vi "Teleop.vi"(10 "Match Info":T1={"Autonomous Elapsed Seconds"=0.0, "TeleOp Elapsed Seconds"=0.0, "Disabled Elapsed Seconds"=0.0, "Visited Autonomous"=FALSE, "Visited TeleOp"=FALSE, "Visited Disabled"=FALSE, "Autonomous Settings"={"Autonomous Style"=enum."Independent", "VI Refnum"=refnum}}, 11 "Call Context":T2) -> ()   [LabVIEW 2013]
doc: "This VI is called for each TeleOp packet received from the DS where the robot is not disabled. It is often used to read from the joysticks and update I/O or to update setpoints for timed control loops. It should complete and return within 20 milliseconds or it may miss DS packets."
uses:
  Robot Global Data.vi
  <vilib>/Rock Robotics/WPI/DriverStation/DriverStationLCD/WPI_DriverStationLCDLCDLine.ctl
  <vilib>/Rock Robotics/WPI/RobotDrive/WPI_RobotDriveArcadeDrive_Standard(NoSaturation).vi
  <vilib>/Rock Robotics/WPI/Solenoid/Deprecated/WPI_SolenoidSetBool.vi
  <vilib>/Rock Robotics/WPI/DriverStation/WPI_DriverStationMatch Info.ctl
  <vilib>/Rock Robotics/WPI/DriverStation/WPI_DriverStationDerivedRobotMode.ctl
panel:
  out "Numeric 1":dbl(slide) scale=0.0..100.0
  out "Boolean 2":bool
  out "Boolean 1":bool
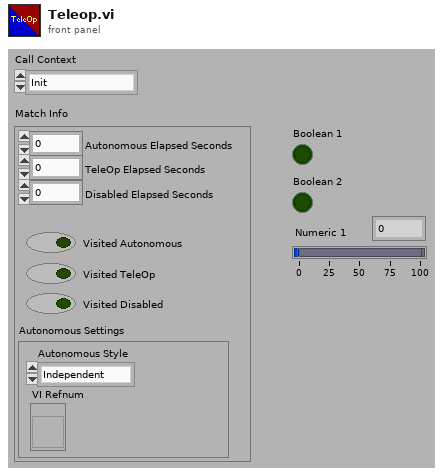
[diagram p1: front panel]
types:
  T1 = typedef "WPI_DriverStationMatch Info.ctl" = cluster{"Autonomous Elapsed Seconds":dbl, "TeleOp Elapsed Seconds":dbl, "Disabled Elapsed Seconds":dbl, "Visited Autonomous":bool, "Visited TeleOp":bool, "Visited Disabled":bool, "Autonomous Settings":cluster{"Autonomous Style":enum16{"Iterative", "Independent"}, "VI Refnum":refnum<vi>}}
  T2 = typedef "WPI_DriverStationDerivedRobotMode.ctl" = enum16{"Init", "Execute", "Stop"}
  T3 = typedef "WPI_DriverStationLCDLCDLine.ctl" = enum16{"Main - Line 1", "User - Line 2", "User - Line 3", "User - Line 4", "User - Line 5", "User - Line 6"}
  T4 = typedef "WPI_DigitalInputDevRef.ctl" = cluster{"DevStatus":errorcluster, "DIO Channel":T5, "Digital Module":T6}
  T5 = typedef "FPGA_DIOChannel.ctl" = enum8{"DIO 1", "DIO 2", "DIO 3", "DIO 4", "DIO 5", "DIO 6", "DIO 7", "DIO 8", "DIO 9", "DIO 10", "DIO 11", "DIO 12", "DIO 13", "DIO 14", "Invalid"}
  T6 = typedef "FPGA_TypedefDigitalModule.ctl" = enum16{"Digital Module 1", "Digital Module 2"}
  T7 = typedef "WPI_JoystickDevRef.ctl" = cluster{"Device":T8}
  T8 = typedef "WPI_JoystickDeviceEnum.ctl" = enum16{"USB 1", "USB 2", "USB 3", "USB 4", "Kinect 1", "Kinect 2"}
  T9 = typedef "WPI_JoystickButtonState.ctl" = cluster{"Button 1":bool, "Button 2":bool, "Button 3":bool, "Button 4":bool, "Button 5":bool, "Button 6":bool, "Button 7":bool, "Button 8":bool, "Button 9":bool, "Button 10":bool, "Button 11":bool, "Button 12":bool}
  T10 = cluster{"axis 1 (x)":dbl, "axis 2 (y)":dbl, "axis 3 (throttle)":dbl, "axis 4":dbl, "axis 5":dbl, "axis 6":dbl}
  T11 = typedef "WPI_MotorControlDeviceRef.ctl" = cluster{"DeviceStatus":errorcluster, "Type":enum16{"PWM", "CAN"}, "PWM":cluster{"Digital Module":T6, "PWM Channel":T12, "DeadBand":T13}, "CAN":cluster{"Device Number":u8, "Control Mode":T14, "Semaphore":T15, "Max Vout":dbl}, "Invert":bool, "TransformRef":T16, "InvTransformRef":T16}
  T12 = typedef "FPGA_DIOPWMChannel.ctl" = enum8{"PWM 1", "PWM 2", "PWM 3", "PWM 4", "PWM 5", "PWM 6", "PWM 7", "PWM 8", "PWM 9", "PWM 10", "Invalid"}
  T13 = typedef "WPI_PWMDeadband.ctl" = cluster{"Name":string, "maxPositivePwm":i32, "minPositivePwm":i32, "centerPwm":i32, "maxNegativePwm":i32, "minNegativePwm":i32, "angularRange":u16}
  T14 = typedef "WPI_CANJaguar_ControlMode.ctl" = enum8{"Percent VBus", "Current", "Speed", "Position", "Voltage"}
  T15 = typedef "Semaphore RefNum" = refnum<k1>
  T16 = typedef "WPI_PWMTransform_ConPane.ctl" = refnum<vi>
  T17 = typedef "WPI_SolenoidDevRef.ctl" = cluster{"DevStatus":errorcluster, "Solenoid Module":T18, "Forward Solenoid Channel":T19, "Reverse Solenoid Channel":T19}
  T18 = typedef "FPGA_TypedefSolenoidModule.ctl" = enum16{"Solenoid Module 1", "Solenoid Module 2"}
  T19 = typedef "WPI_SolenoidChannel.ctl" = enum8{"Solenoid 1", "Solenoid 2", "Solenoid 3", "Solenoid 4", "Solenoid 5", "Solenoid 6", "Solenoid 7", "Solenoid 8", "Invalid"}
  T20 = typedef "WPI_RobotDriveDevRef.ctl" = cluster{"DevStatus":errorcluster, "Motors[]":T11[], "Square Inputs":bool, "Max Output":dbl, "Isochronous":bool}
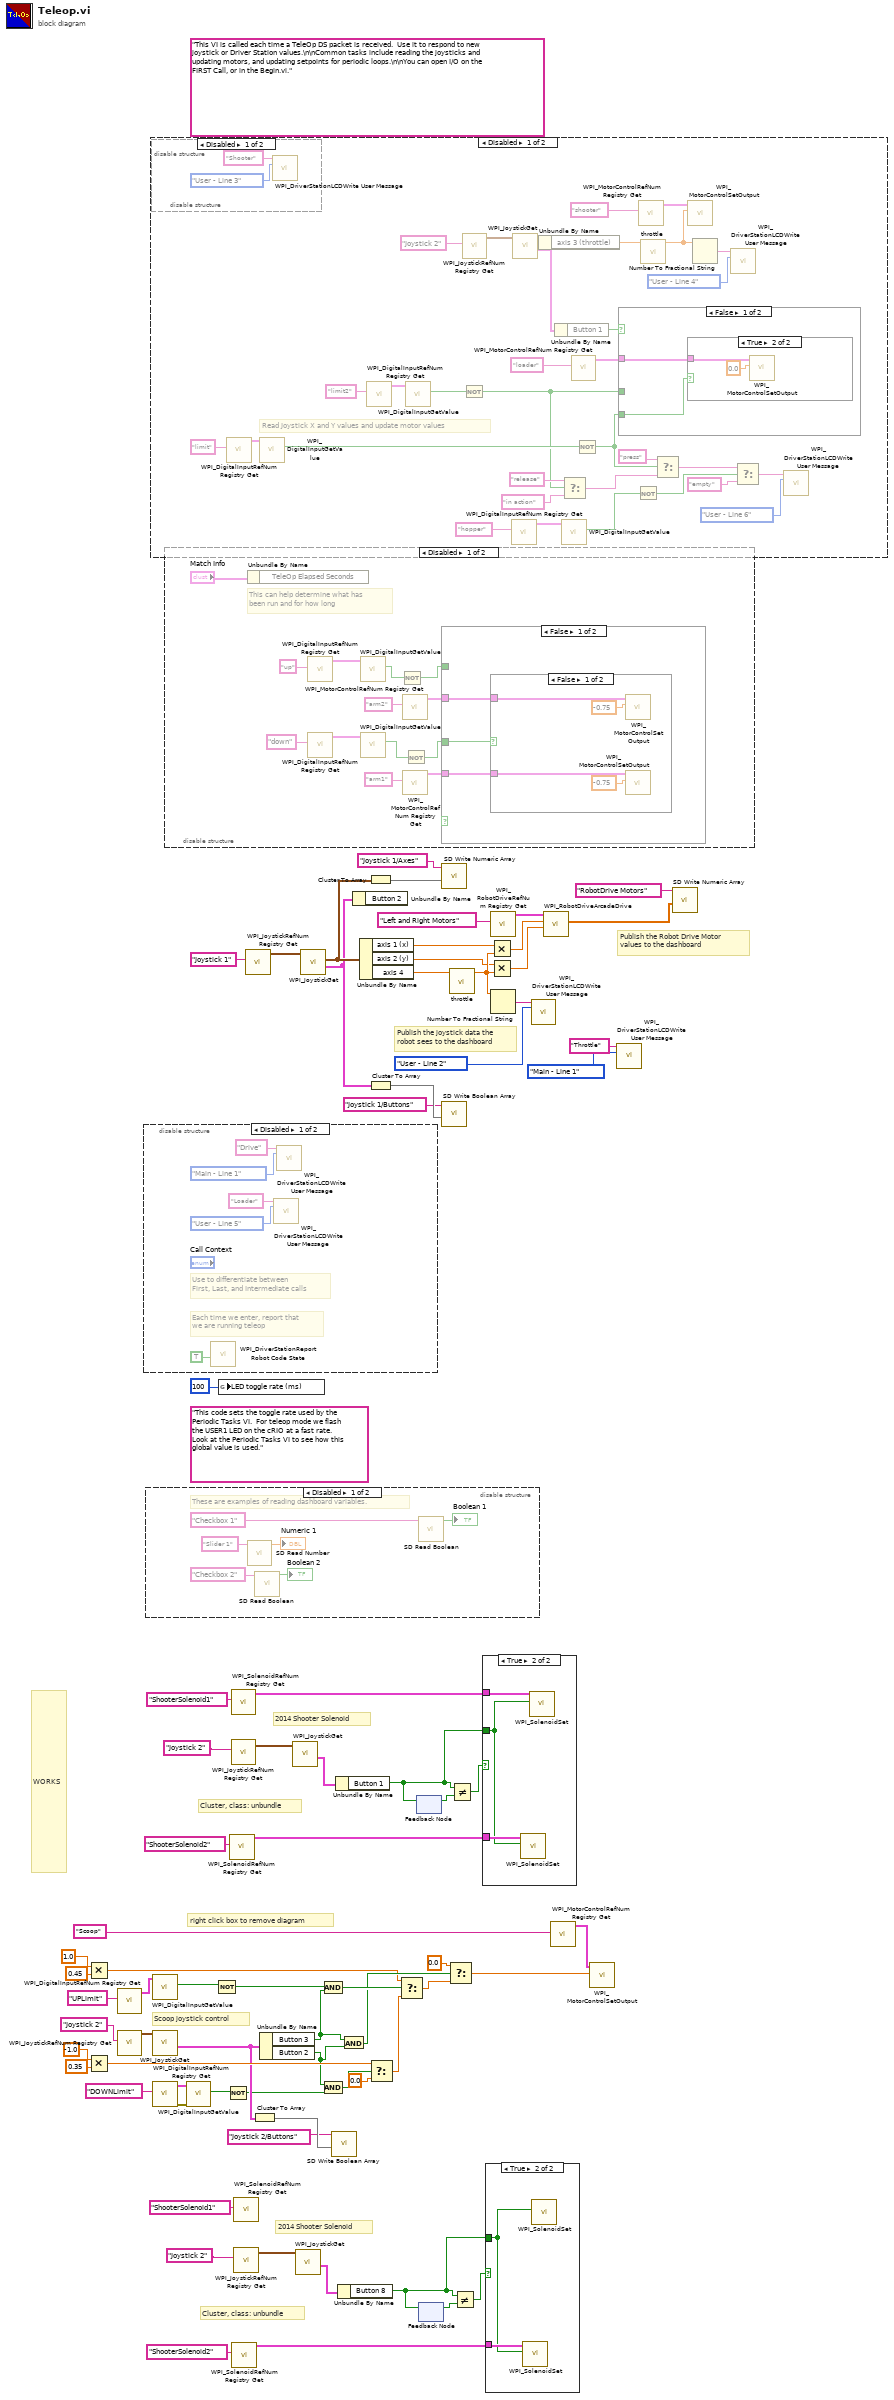
[diagram p0: block diagram]
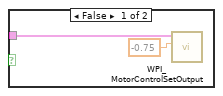
[diagram p3: hidden frame]
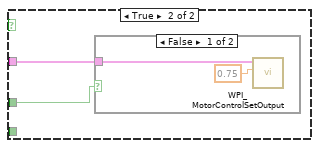
[diagram p4: hidden frame]
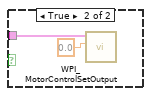
[diagram p5: hidden frame]
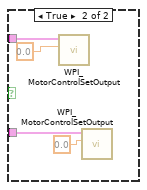
[diagram p11: hidden frame]
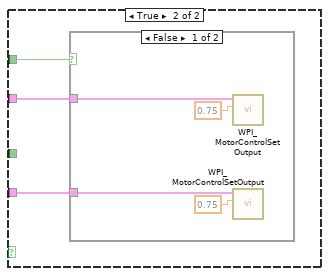
[diagram p12: hidden frame]
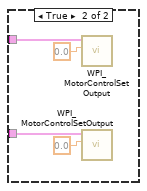
[diagram p13: hidden frame]
diagram:
  (unwired) "This code sets the toggle rate used by the Periodic Tasks VI.  For teleop mode we flash the USER1 LED on the cRIO at a fast rate.  Look at the Periodic Tasks VI to see how this global value is used."
  (unwired) "This VI is called each time a TeleOp DS packet is received.  Use it to respond to new joystick or Driver Station values.\n\nCommon tasks include reading the joysticks and updating motors, and updating setpoints for periodic loops.\n\nYou can open I/O on the FIRST Call, or in the Begin.vi."
  # "2014 Shooter Solenoid"
  # "Cluster, class: unbundle"
  # "right click box to remove diagram"
  # "Scoop joystick control"
  # "WORKS"
  # "2014 Shooter Solenoid"
  # "Cluster, class: unbundle"
  # "Publish the Robot Drive Motor\nvalues to the dashboard"
  # "Publish the joystick data the\nrobot sees to the dashboard"
  n1 = Multiply(x=1.0, y=0.45) -> (x*y=w22:dbl)
  n2 = Multiply(x=-1.0, y=0.35) -> (x*y=w23:dbl)
  n3 = call <vilib>:"WPI_DigitalInputRefNum Registry Get.vi"("refnum name"="UPLimit") -> ("DigitalInputDevRef"=w37:T4)  [unwired: 9 in, 1 out]
  n4 = call <vilib>:"WPI_JoystickRefNum Registry Get.vi"("refnum name"="Joystick 2") -> ("JoystickDevRef"=w40:T7)  [unwired: 9 in, 1 out]
  n5 = disable-structure shown="Disabled" {
    frame Disabled {
      # "Each time we enter, report that\nwe are running teleop"
      # "Use to differentiate between\nFirst, Last, and Intermediate calls"
      n6 = call <vilib>:"WPI_DriverStationReport Robot Code State.vi"("TeleOp"=TRUE ("Autonomous")) -> ()  [unwired: 10 in, 1 out]
      n7 = call <vilib>:"WPI_DriverStationLCDWrite User Message.vi"("line text"="Loader", "line"=WPI_DriverStationLCDLCDLine."User - Line 5") -> ()  [unwired: 13 in, 1 out]
      n8 = call <vilib>:"WPI_DriverStationLCDWrite User Message.vi"("line text"="Drive", "line"=WPI_DriverStationLCDLCDLine."Main - Line 1") -> ()  [unwired: 13 in, 1 out]
    }
    frame Enabled {
    }
  }
  n9 = disable-structure shown="Disabled" {
    frame Disabled {
      # "These are examples of reading dashboard variables."
      n10 = call <vilib>:"SD Read Number.vi"("Name"="Slider 1" ("refnum name")) -> ("Numeric"=→"Numeric 1":dbl)  [unwired: 8 in, 2 out]
      n11 = call <vilib>:"SD Read Boolean.vi"("Name"="Checkbox 2" ("refnum name")) -> ("Boolean"=→"Boolean 2":bool)  [unwired: 8 in, 2 out]
      n12 = call <vilib>:"SD Read Boolean.vi"("Name"="Checkbox 1" ("refnum name")) -> ("Boolean"=→"Boolean 1":bool)  [unwired: 8 in, 2 out]
    }
    frame Enabled {
    }
  }
  n13 = disable-structure shown="Disabled" {
    frame Disabled {
      # "Read Joystick X and Y values and update motor values"
      n14 = disable-structure shown="Disabled" {
        frame Disabled {
          n15 = call <vilib>:"WPI_DriverStationLCDWrite User Message.vi"("line text"="Shooter", "line"=WPI_DriverStationLCDLCDLine."User - Line 3") -> ()  [unwired: 13 in, 1 out]
        }
        frame Enabled {
        }
      }
      n16 = call <vilib>:"WPI_DigitalInputRefNum Registry Get.vi"("refnum name"="limit") -> ("DigitalInputDevRef"=w115:T4)  [unwired: 9 in, 1 out]
      n17 = call <vilib>:"WPI_DigitalInputGetValue.vi"("DigitalInputDevRef"=w115) -> ("Value"=w109:bool)  [unwired: 8 in, 2 out]
      n18 = call <vilib>:"WPI_DigitalInputRefNum Registry Get.vi"("refnum name"="limit2") -> ("DigitalInputDevRef"=w111:T4)  [unwired: 9 in, 1 out]
      n19 = call <vilib>:"WPI_DigitalInputGetValue.vi"("DigitalInputDevRef"=w111) -> ("Value"=w110:bool)  [unwired: 8 in, 2 out]
      n20 = Not(x=w110) -> (.not. x?=w103:bool)
      n21 = call <vilib>:"WPI_JoystickRefNum Registry Get.vi"("refnum name"="Joystick 2") -> ("JoystickDevRef"=w101:T7)  [unwired: 1 in, 9 out]
      n22 = call <vilib>:"WPI_DigitalInputRefNum Registry Get.vi"("refnum name"="hopper") -> ("DigitalInputDevRef"=w91:T4)  [unwired: 9 in, 1 out]
      n23 = call <vilib>:"WPI_JoystickGet.vi"("JoystickDevRef"=w101) -> ("Buttons"=w98:T9, "Axes"=w99:T10)  [unwired: 1 in, 4 out]
      n24 = Unbundle By Name(w99) -> ("axis 3 (throttle)"=w97:dbl)
      n25 = Unbundle By Name(w98) -> ("Button 1"=w94:bool)
      n26 = call <vilib>:"WPI_DigitalInputGetValue.vi"("DigitalInputDevRef"=w91) -> ("Value"=w90:bool)  [unwired: 8 in, 2 out]
      n27 = Select(t="release", s=w103, f="in action") -> (s? t:f=w108:string)
      n28 = call <vilib>:"WPI_MotorControlRefNum Registry Get.vi"("refnum name"="loader") -> ("MotorControlDevRef"=w102:T11)  [unwired: 9 in, 1 out]
      n29 = Not(x=w109) -> (.not. x?=w104:bool)
      n30 = case shown="False" w94 {
        tunnel: w102 -> [w119 w125]
        tunnel: w103 -> [_ w126]
        tunnel: w104 -> [w120 _]
        frame False {
          n31 = case shown="True" w120 {
            tunnel: w119 -> [w121 w123]
            frame False {
              n32 = call <vilib>:"WPI_MotorControlSetOutput.vi"("Output"=-0.75, "MotorControlDevRef"=w121) -> ()  [unwired: 7 in, 3 out]
            }
            frame True {
              n33 = call <vilib>:"WPI_MotorControlSetOutput.vi"("Output"=0.0, "MotorControlDevRef"=w123) -> ()  [unwired: 7 in, 3 out]
            }
          }
        }
        frame True {
          n34 = case shown="False" w126 {
            tunnel: w125 -> [w128 w130]
            frame False {
              n35 = call <vilib>:"WPI_MotorControlSetOutput.vi"("Output"=0.75, "MotorControlDevRef"=w128) -> ()  [unwired: 7 in, 3 out]
            }
            frame True {
              n36 = call <vilib>:"WPI_MotorControlSetOutput.vi"("Output"=0.0, "MotorControlDevRef"=w130) -> ()  [unwired: 7 in, 3 out]
            }
          }
        }
      }
      n37 = Not(x=w90) -> (.not. x?=w87:bool)
      n38 = call <vilib>:"WPI_MotorControlRefNum Registry Get.vi"("refnum name"="shooter") -> ("MotorControlDevRef"=w118:T11)  [unwired: 9 in, 1 out]
      n39 = call "throttle.vi"("x"=w97) -> ("x/y"=w93:dbl)  [unwired: 10 in]
      n40 = Select(t="press", s=w104, f=w108) -> (s? t:f=w89:string)
      n41 = call <vilib>:"WPI_MotorControlSetOutput.vi"("Output"=w93, "MotorControlDevRef"=w118) -> ()  [unwired: 7 in, 3 out]
      n42 = Number To Fractional String(number=w93) -> (F-format string=w96:string)  [unwired: 3 in]
      n43 = call <vilib>:"WPI_DriverStationLCDWrite User Message.vi"("line text"=w96, "line"=WPI_DriverStationLCDLCDLine."User - Line 4") -> ()  [unwired: 13 in, 1 out]
      n44 = Select(t=w89, s=w87, f="empty") -> (s? t:f=w88:string)
      n45 = call <vilib>:"WPI_DriverStationLCDWrite User Message.vi"("line text"=w88, "line"=WPI_DriverStationLCDLCDLine."User - Line 6") -> ()  [unwired: 13 in, 1 out]
    }
    frame Enabled {
    }
  }
  n46 = call <vilib>:"WPI_DigitalInputGetValue.vi"("DigitalInputDevRef"=w37) -> ("Value"=w13:bool)  [unwired: 8 in, 2 out]
  n47 = call <vilib>:"WPI_JoystickGet.vi"("JoystickDevRef"=w40) -> ("Buttons"=w16:T9)  [unwired: 4 in, 2 out]
  n48 = call <vilib>:"WPI_DigitalInputRefNum Registry Get.vi"("refnum name"="DOWNLimit") -> ("error out"=w39:errorcluster, "DigitalInputDevRef"=w38:T4)  [unwired: 9 in]
  n49 = disable-structure shown="Disabled" {
    frame Disabled {
      # "This can help determine what has\nbeen run and for how long"
      n50 = Unbundle By Name("Match Info") -> ()  [unwired: 1 out]
      n51 = call <vilib>:"WPI_DigitalInputRefNum Registry Get.vi"("refnum name"="up") -> ("DigitalInputDevRef"=w144:T4)  [unwired: 9 in, 1 out]
      n52 = call <vilib>:"WPI_DigitalInputRefNum Registry Get.vi"("refnum name"="down") -> ("DigitalInputDevRef"=w143:T4)  [unwired: 9 in, 1 out]
      n53 = call <vilib>:"WPI_DigitalInputGetValue.vi"("DigitalInputDevRef"=w144) -> ("Value"=w136:bool)  [unwired: 8 in, 2 out]
      n54 = call <vilib>:"WPI_DigitalInputGetValue.vi"("DigitalInputDevRef"=w143) -> ("Value"=w134:bool)  [unwired: 8 in, 2 out]
      n55 = Not(x=w136) -> (.not. x?=w135:bool)
      n56 = call <vilib>:"WPI_MotorControlRefNum Registry Get.vi"("refnum name"="arm2") -> ("MotorControlDevRef"=w139:T11)  [unwired: 9 in, 1 out]
      n57 = call <vilib>:"WPI_MotorControlRefNum Registry Get.vi"("refnum name"="arm1") -> ("MotorControlDevRef"=w140:T11)  [unwired: 9 in, 1 out]
      n58 = Not(x=w134) -> (.not. x?=w133:bool)
      n59 = case shown="False" {
        selector: _ -> [_ _]
        tunnel: w135 -> [_ w159]
        tunnel: w133 -> [w148 _]
        tunnel: w140 -> [w147 w158]
        tunnel: w139 -> [w146 w157]
        frame False {
          n60 = case shown="False" w148 {
            tunnel: w147 -> [w150 w155]
            tunnel: w146 -> [w149 w154]
            frame False {
              n61 = call <vilib>:"WPI_MotorControlSetOutput.vi"("Output"=-0.75, "MotorControlDevRef"=w149) -> ()  [unwired: 7 in, 3 out]
              n62 = call <vilib>:"WPI_MotorControlSetOutput.vi"("Output"=-0.75, "MotorControlDevRef"=w150) -> ()  [unwired: 7 in, 3 out]
            }
            frame True {
              n63 = call <vilib>:"WPI_MotorControlSetOutput.vi"("Output"=0.0, "MotorControlDevRef"=w154) -> ()  [unwired: 7 in, 3 out]
              n64 = call <vilib>:"WPI_MotorControlSetOutput.vi"("Output"=0.0, "MotorControlDevRef"=w155) -> ()  [unwired: 7 in, 3 out]
            }
          }
        }
        frame True {
          n65 = case shown="False" w159 {
            tunnel: w158 -> [w161 w165]
            tunnel: w157 -> [w160 w164]
            frame False {
              n66 = call <vilib>:"WPI_MotorControlSetOutput.vi"("Output"=0.75, "MotorControlDevRef"=w160) -> ()  [unwired: 7 in, 3 out]
              n67 = call <vilib>:"WPI_MotorControlSetOutput.vi"("Output"=0.75, "MotorControlDevRef"=w161) -> ()  [unwired: 7 in, 3 out]
            }
            frame True {
              n68 = call <vilib>:"WPI_MotorControlSetOutput.vi"("Output"=0.0, "MotorControlDevRef"=w164) -> ()  [unwired: 7 in, 3 out]
              n69 = call <vilib>:"WPI_MotorControlSetOutput.vi"("Output"=0.0, "MotorControlDevRef"=w165) -> ()  [unwired: 7 in, 3 out]
            }
          }
        }
      }
    }
    frame Enabled {
    }
  }
  n70 = call <vilib>:"WPI_DigitalInputGetValue.vi"("error in (no error)"=w39, "DigitalInputDevRef"=w38) -> ("Value"=w15:bool)  [unwired: 7 in, 2 out]
  n71 = Not(x=w13) -> (.not. x?=w12:bool)
  n72 = global write "Robot Global Data.vi" "LED toggle rate (ms)"(u32 100 ("LED ms toggle rate")) -> ()
  n73 = Not(x=w15) -> (.not. x?=w14:bool)
  n74 = call <vilib>:"WPI_SolenoidRefNum Registry Get.vi"("refnum name"="ShooterSolenoid2") -> ("SolenoidDevRef"=w47:T17)  [unwired: 9 in, 1 out]
  n75 = call <vilib>:"WPI_SolenoidRefNum Registry Get.vi"("refnum name"="ShooterSolenoid1") -> ("SolenoidDevRef"=w52:T17)  [unwired: 9 in, 1 out]
  n76 = call <vilib>:"WPI_JoystickRefNum Registry Get.vi"("refnum name"="Joystick 2") -> ("JoystickDevRef"=w51:T7)  [unwired: 9 in, 1 out]
  n77 = call <vilib>:"WPI_SolenoidRefNum Registry Get.vi"("refnum name"="ShooterSolenoid2") -> ("SolenoidDevRef"=w4:T17)  [unwired: 9 in, 1 out]
  n78 = call <vilib>:"WPI_SolenoidRefNum Registry Get.vi"("refnum name"="ShooterSolenoid1") -> ()  [unwired: 9 in, 2 out]
  n79 = call <vilib>:"WPI_JoystickRefNum Registry Get.vi"("refnum name"="Joystick 2") -> ("JoystickDevRef"=w8:T7)  [unwired: 9 in, 1 out]
  n80 = call <vilib>:"WPI_JoystickRefNum Registry Get.vi"("refnum name"="Joystick 1") -> ("JoystickDevRef"=w72:T7)  [unwired: 1 in, 9 out]
  n81 = Cluster To Array(cluster=w16) -> (array=w18:bool[])
  n82 = Unbundle By Name(w16) -> ("Button 3"=w20:bool, "Button 2"=w19:bool)
  n83 = call <vilib>:"WPI_JoystickGet.vi"("JoystickDevRef"=w51) -> ("Buttons"=w49:T9)  [unwired: 4 in, 2 out]
  n84 = call <vilib>:"WPI_JoystickGet.vi"("JoystickDevRef"=w8) -> ("Buttons"=w6:T9)  [unwired: 4 in, 2 out]
  n85 = call <vilib>:"WPI_JoystickGet.vi"("JoystickDevRef"=w72) -> ("Buttons"=w54:T9, "Axes"=w68:T10)  [unwired: 1 in, 4 out]
  n86 = And(x=w12, y=w20) -> (x .and. y?=w34:bool)
  n87 = And(x=w19, y=w14) -> (x .and. y?=w33:bool)
  n88 = call <vilib>:"SD Write Boolean Array.vi"("Boolean Array"=w18, "Name"="Joystick 2/Buttons") -> ()  [unwired: 8 in, 2 out]
  n89 = Unbundle By Name(w49) -> ("Button 1"=w44:bool)
  n90 = Unbundle By Name(w6) -> ("Button 8"=w1:bool)
  n91 = And(x=w20, y=w19) -> (x .and. y?=w29:bool)
  n92 = Unbundle By Name(w54) -> ()  [unwired: 1 out]
  n93 = Unbundle By Name(w68) -> ("axis 1 (x)"=w61:dbl, "axis 2 (y)"=w55:dbl, "axis 4"=w63:dbl)
  n94 = Cluster To Array(cluster=w68) -> (array=w67:dbl[])
  n95 = Cluster To Array(cluster=w54) -> (array=w70:bool[])
  n96 = Select(t=w23, s=w33, f=0.0) -> (s? t:f=w27:dbl)
  n97 = Select(t=w22, s=w34, f=w27) -> (s? t:f=w31:dbl)
  n98 = feedback-in #1(w44) -> ()
  n99 = feedback #1() -> (w45:bool)  [unwired: 1 in]
  n100 = feedback #2() -> (w2:bool)  [unwired: 1 in]
  n101 = feedback-in #2(w1) -> ()
  n102 = call <vilib>:"SD Write Numeric Array.vi"("Numeric Array"=w67, "Name"="Joystick 1/Axes") -> ()  [unwired: 8 in, 2 out]
  n103 = call <vilib>:"SD Write Boolean Array.vi"("Boolean Array"=w70, "Name"="Joystick 1/Buttons") -> ()  [unwired: 8 in, 2 out]
  n104 = Select(t=0.0, s=w29, f=w31) -> (s? t:f=w21:dbl)
  n105 = call "throttle.vi"("x"=w63) -> ("x/y"=w58:dbl)  [unwired: 10 in]
  n106 = Not Equal?(x=w44, y=w45) -> (x != y?=w46:bool)
  n107 = Not Equal?(x=w1, y=w2) -> (x != y?=w3:bool)
  n108 = case shown="True" w46 {
    tunnel: w52 -> [_ w170]
    tunnel: w47 -> [_ w169]
    tunnel: w44 -> [_ w168]
    frame False {
    }
    frame True {
      n109 = call-poly <vilib>:"WPI_SolenoidSet.vi"("Value"=w168, "SolenoidDevRef"=w169) -> ()  [unwired: 8 in, 2 out]
      n110 = call-poly <vilib>:"WPI_SolenoidSet.vi"("Value"=w168, "SolenoidDevRef"=w170) -> ()  [unwired: 8 in, 2 out]
    }
  }
  n111 = case shown="True" w3 {
    tunnel: w4 -> [_ w172]
    tunnel: w1 -> [_ w171]
    frame False {
    }
    frame True {
      n112 = call-poly <vilib>:"WPI_SolenoidSet.vi"("Value"=w171, "SolenoidDevRef"=w172) -> ()  [unwired: 8 in, 2 out]
      n113 = call-poly <vilib>:"WPI_SolenoidSet.vi"("Value"=w171) -> ()  [unwired: 9 in, 2 out]
    }
  }
  n114 = Multiply(x=w61, y=w58) -> (x*y=w60:dbl)
  n115 = Multiply(x=w55, y=w58) -> (x*y=w62:dbl)
  n116 = call <vilib>:"WPI_RobotDriveRefNum Registry Get.vi"("refnum name"="Left and Right Motors") -> ("RobotDriveDevRef"=w56:T20)  [unwired: 1 in, 9 out]
  n117 = Number To Fractional String(number=w58) -> (F-format string=w59:string)  [unwired: 3 in]
  n118 = call <vilib>:"WPI_DriverStationLCDWrite User Message.vi"("line text"=w59, "line"=WPI_DriverStationLCDLCDLine."User - Line 2") -> ()  [unwired: 13 in, 1 out]
  n119 = call-poly <vilib>:"WPI_RobotDriveArcadeDrive.vi"("Y axis value"=w62, "X axis value"=w60, "RobotDriveDevRef"=w56) -> ("Motor Values"=w64:dbl[])  [unwired: 6 in, 2 out]
  n120 = call <vilib>:"WPI_MotorControlRefNum Registry Get.vi"("refnum name"="Scoop") -> ("MotorControlDevRef"=w42:T11)  [unwired: 9 in, 1 out]
  n121 = call <vilib>:"WPI_MotorControlSetOutput.vi"("Output"=w21, "MotorControlDevRef"=w42) -> ()  [unwired: 7 in, 3 out]
  n122 = call <vilib>:"WPI_DriverStationLCDWrite User Message.vi"("line text"="Throttle", "line"=WPI_DriverStationLCDLCDLine."Main - Line 1") -> ()  [unwired: 13 in, 1 out]
  n123 = call <vilib>:"SD Write Numeric Array.vi"("Numeric Array"=w64, "Name"="RobotDrive Motors") -> ()  [unwired: 8 in, 2 out]
